vi "latch variable panel test.vi"() -> ()   [LabVIEW 2010]
panel:
  out "num presses":i16
  in  "stop":bool
  in  "OK Button":bool
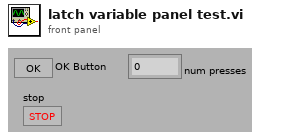
[diagram p1: front panel]
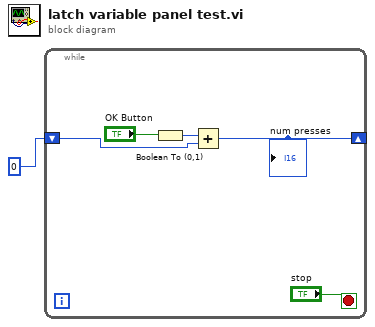
[diagram p0: block diagram]
diagram:
  n1 = while {
    shift-right: [w3] -> _
    shift-left: i16 0 ("Numeric") -> [w2]
    stop <- "stop" stop-if-true
    n2 = Boolean To (0,1)(Boolean="OK Button") -> (0, 1=w4:i16)
    n3 = Add(x=w4, y=w2) -> (x+y=w3:i16)
    "num presses" <- w3
  }
